vi "Initialize Default.vi"(8 "error in (no error)":errorcluster, 11 "UDP Tx Transfer Configuration in":refnum<class "UDP Transfer Tx Configuration.lvclass">) -> (0 "error out":errorcluster, 3 "UDP Tx Transfer Configuration out":refnum<class "UDP Transfer Tx Configuration.lvclass">)   [LabVIEW 2017, in "UDP.lvlib" / "UDP Transfer Tx Configuration.lvclass"]
uses:
  UDP Transfer Tx Configuration.lvclass
  UDP Transfer Tx Configuration.lvclass/UDP Transfer Tx Configuration.ctl
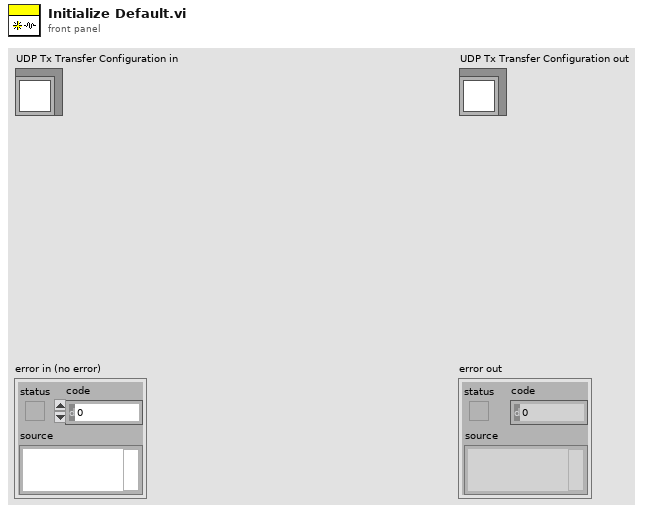
[diagram p1: front panel]
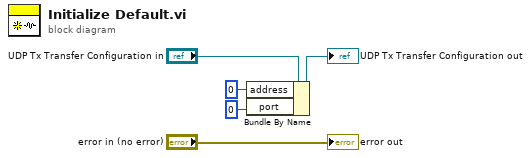
[diagram p0: block diagram]
diagram:
  n1 = Bundle By Name(cluster="UDP Tx Transfer Configuration in", "address"=u32 0 ("tx transfer settings.address"), "port"=u16 0 ("tx transfer settings.port")) -> (→"UDP Tx Transfer Configuration out":refnum<class "UDP Transfer Tx Configuration.lvclass">)
  "error out" <- "error in (no error)"
